vi "Send UI Limits.vi"(10 "Data":variant, 11 "CtlRef":refnum<vi>) -> ()   [LabVIEW 2018, in "Messaging.lvlib"]
doc: "Convenience wrapper for sending value change events from the UI to the audio processing loop."
uses:
  Messaging.lvlib
  Message Cluster.ctl
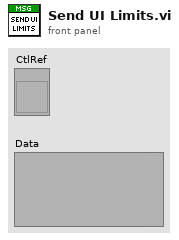
[diagram p1: front panel]
types:
  T1 = typedef "Messaging.lvlib/Message Cluster.ctl" = cluster{"Event":string, "Source":string, "Target":string, "Data":variant}
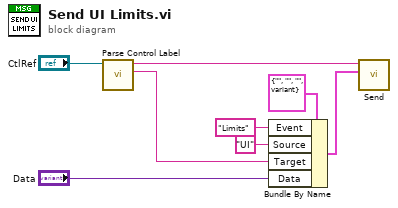
[diagram p0: block diagram]
diagram:
  n1 = call "Parse Control Label.vi"("CtlRef"="CtlRef") -> ("Value Name"=w4:string, "Queue Name"=w5:string)  [unwired: 9 in]
  n2 = Bundle By Name(cluster=T1 {"Event"="", "Source"="", "Target"="", "Data"=variant} ("Message"), "Event"="Limits" ("Type"), "Source"="UI" ("Event"), "Target"=w4, "Data"="Data") -> (w6:T1)
  n3 = call "Send.vi"("Message"=w6, "Queue Name"=w5) -> ()  [unwired: 9 in, 1 out]
